vi "Configure Branch Delta.vi"(6 "Measure Block (0)":u32, 7 "Target Difference (0)":dbl, 8 "error in (no error)":errorcluster, 9 "Branch To Block (0)":u32, 10 "Block Number (1)":u32=1, 11 "VISA resource name":refnum<visa-resource-name>) -> (0 "error out":errorcluster, 3 "VISA resource name out":refnum<visa-resource-name>)   [LabVIEW 2023, in "Keithley DMM6500 DAQ6500 Series.lvlib"]
doc: "Defines a trigger model block that goes to a specified block if the difference of two measurements meets preset criteria.\nThis block calculates the difference between the last two measurements from a measure or digitize block. It subtracts the most recent measurement from the previous measurement."
uses:
  <instrlib>/Keithley DMM6500 DAQ6500 Series/Keithley DMM6500 DAQ6500 Series.lvlib
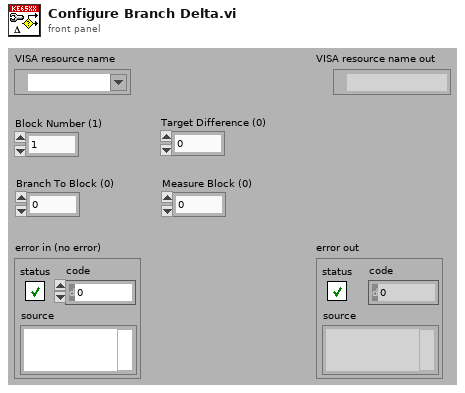
[diagram p1: front panel]
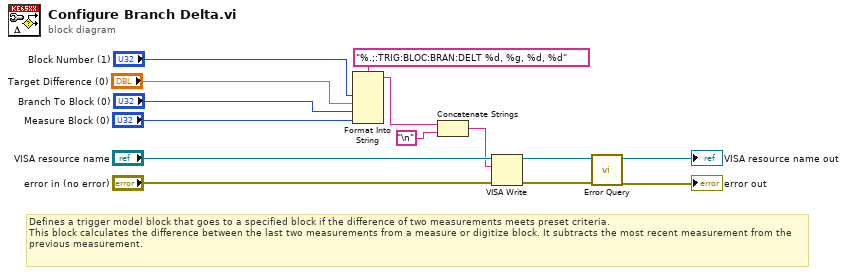
[diagram p0: block diagram]
diagram:
  # "Defines a trigger model block that goes to a specified block if the difference of two measurements meets preset criteria.\nThis block calculates the difference between the last two measurements from a measure or digitize block. It subtracts the most recent measurement from the previous measurement."
  n1 = Format Into String(format string="%.;:TRIG:BLOC:BRAN:DELT %d, %g, %d, %d", "Block Number (1)", "Target Difference (0)", "Branch To Block (0)", "Measure Block (0)") -> (resulting string=w3:string)  [unwired: 2 in, 1 out]
  n2 = Concatenate Strings(w3, "\n") -> (w5:string)
  n3 = VISA Write(VISA resource name="VISA resource name", write buffer=w5, error in (no error)="error in (no error)") -> (VISA resource name out=w9:refnum<visa-resource-name>, error out=w8:errorcluster)  [unwired: 1 out]
  n4 = call <instrlib>:"Error Query.vi"("error in (no error)"=w8, "VISA resource name"=w9) -> ("error out"=→"error out":errorcluster, "VISA resource name out"=→"VISA resource name out":refnum<visa-resource-name>)  [unwired: 6 in, 2 out]
